vi "TesterModule.Init.vi"(8 "error in (no error)":errorcluster, 9 "JQMHStartup in":refnum<class "JQMHStartup.lvclass">, 11 "TesterModule in":refnum<class "TesterModule.lvclass">) -> (0 "error out":errorcluster, 1 "JQMHStartup out":refnum<class "JQMHStartup.lvclass">, 2 "TesterModule.Requests":cluster{"Requests":T1, "Requests":T2}, 3 "TesterModule out":refnum<class "TesterModule.lvclass">, 4 "StartupParams":variant, 5 "Event Registration Refnum":refnum<event-registration>)   [LabVIEW 2024, in "TesterModule.lvclass"]
uses:
  TesterModule.lvclass
  JQMHCore/JQMHStartup/JQMHStartup.lvclass
  JQMHCore/Module/StandardRequests.ctl
  JQMHCore/Module/InitialiseArgs.ctl
  JQMHCore/Module/Reply.ctl
  JQMHCore/Module/StopEventArgs.ctl
  JQMHCore/Module/Show Front Panel--Args.ctl
  JQMHCore/Module/Hide Front Panel.ctl
  JQMHCore/Module/Show Block Diagram.ctl
  JQMHCore/Module/Hide Block Diagram--Args.ctl
  Request Events--cluster.ctl
  JQMHCore/Module/JQMHModule.lvclass/JQMHModule.ctl
  TesterModule.lvclass/TesterModule.ctl
  JQMHCore/Shared/JQMHShared.lvlib
  JQMHCore/Module/JQMHModule.lvclass
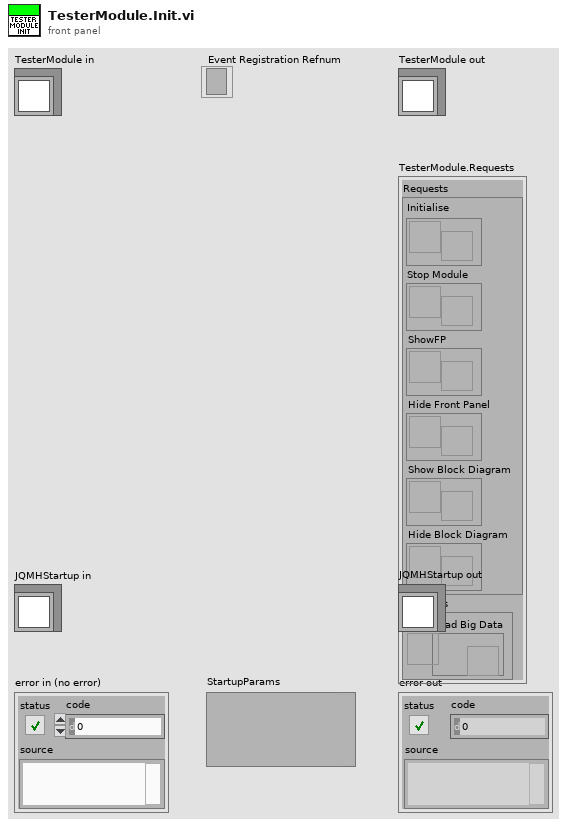
[diagram p1: front panel]
types:
  T1 = typedef "JQMHModule.lvclass/StandardRequests.ctl" = cluster{"Initialise":refnum<user-event>, "Stop Module":refnum<user-event>, "ShowFP":refnum<user-event>, "Hide Front Panel":refnum<user-event>, "Show Block Diagram":refnum<user-event>, "Hide Block Diagram":refnum<user-event>}
  T2 = typedef "TesterModule.lvclass/Request Events--cluster.ctl" = cluster{"Load Big Data":refnum<user-event>}
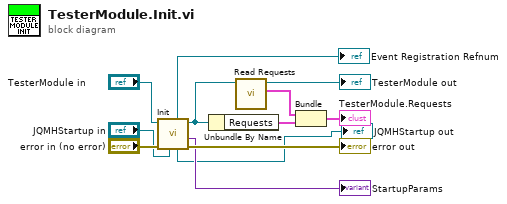
[diagram p0: block diagram]
diagram:
  n1 = call "Init.vi"("JQMHStartup.lvclass"="JQMHStartup in", "error in (no error)"="error in (no error)", "JQMHCore.lvclass"="TesterModule in") -> ("error out"=→"error out":errorcluster, "StartupParams"=→"StartupParams":variant, "JQMHCore out"=w4:refnum<class "TesterModule.lvclass">, "JQMHStartup out"=→"JQMHStartup out":refnum<class "JQMHStartup.lvclass">, "Event Registration Refnum"=→"Event Registration Refnum":refnum<event-registration>)  [unwired: 4 in]
  n2 = Unbundle By Name(w4) -> ("Requests"=w6:T2)
  n3 = call "Read Requests.vi"("JQMHModule in"=w4) -> ("Requests"=w7:T1, "JQMHModule out"=→"TesterModule out":refnum<class "TesterModule.lvclass">)  [unwired: 9 in]
  n4 = Bundle("Requests"=w7, "Requests"=w6) -> (→"TesterModule.Requests":cluster{"Requests":T1, "Requests":T2})  [unwired: 1 in]
